vi "Parse Set Delimiter.vi"(8 "Error In":errorcluster) -> (0 "Error Out":errorcluster)   [LabVIEW 2018, in "Tests.lvlib" / "Parser.lvlib"]
uses:
  Parser.lvlib
  src/Toolkit/Public/Readers/String/String.lvclass
  D:/Users/cfield/Code/Field R&D Services/Mustache/trunk/src/Mustache/Public/Readers/Public/Abstract/Abstract.lvclass
  <vilib>/addons/_JKI Toolkits/Caraya/classes/Test/Test.lvclass
  src/Toolkit/Public/Parser/Parser.lvclass
  <vilib>/addons/_JKI Toolkits/Caraya/classes/Assert/Assert.lvclass
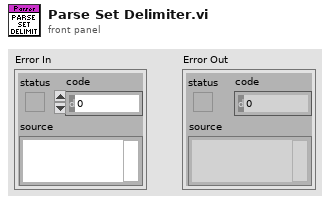
[diagram p1: front panel]
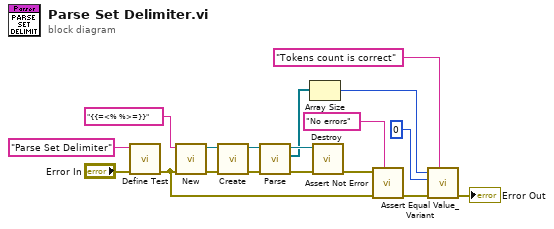
[diagram p0: block diagram]
diagram:
  n1 = call <vilib>:"Define Test.vi"("error in (no error)"="Error In", "Label (VI Title)"="Parse Set Delimiter") -> ("error out"=w9:errorcluster)  [unwired: 9 in]
  n2 = call "New.vi"("Error In"=w9, "String"="{{=<% %>=}}" ("format string")) -> ("Error Out"=w15:errorcluster, "String"=w16:refnum<class "String.lvclass">)  [unwired: 8 in]
  n3 = call "Create.vi"("Error In"=w15, "Reader"=w16) -> ("Error Out"=w14:errorcluster, "Parser"=w13:refnum<class "Parser.lvclass">)  [unwired: 8 in]
  n4 = call "Parse.vi"("Error In"=w14, "Parser In"=w13) -> ("Error Out"=w11:errorcluster, "Tokens"=w3:refnum<class "Abstract.lvclass">[], "Parser Out"=w12:refnum<class "Parser.lvclass">)  [unwired: 7 in]
  n5 = Array Size(array=w3) -> (size(s)=w5:i32)
  n6 = call "Destroy.vi"("Error In"=w11, "Parser"=w12) -> ("Error Out"=w10:errorcluster)  [unwired: 9 in]
  n7 = call <vilib>:"Assert Not Error.vi"("Label"="No errors", "error in (no error)"=w9, "Not Error?"=w10) -> ("error out"=w7:errorcluster)  [unwired: 8 in]
  n8 = call <vilib>:"Assert Equal Value_Variant.vi"("Label"="Tokens count is correct", "error in (no error)"=w7, "Y"=0 ("size(s)"), "X"=w5) -> ("error out"=→"Error Out":errorcluster)  [unwired: 7 in]
